vi "Main On Load Action VI.vi"(8 "error in (no error)":errorcluster, 11 "Device Item Ref in":T1 format="%.0x") -> (0 "error out":errorcluster, 3 "Device Item Ref out":T1 format="%.0x")   [LabVIEW 2019, in "Engine Simulation Toolkit System Explorer.lvlib"]
uses:
  Engine Simulation Toolkit System Explorer.lvlib
  <vilib>/NI VeriStand/Custom Device API/Custom Device Item Ref.ctl
  NationalInstruments.VeriStand.SystemDefinitionAPI
  Shared/Constants and GUIDs.vi
  <vilib>/NI VeriStand/Custom Device API/Custom Device API.lvlib
  Shared/Engine Simulation Toolkit Shared.lvlib
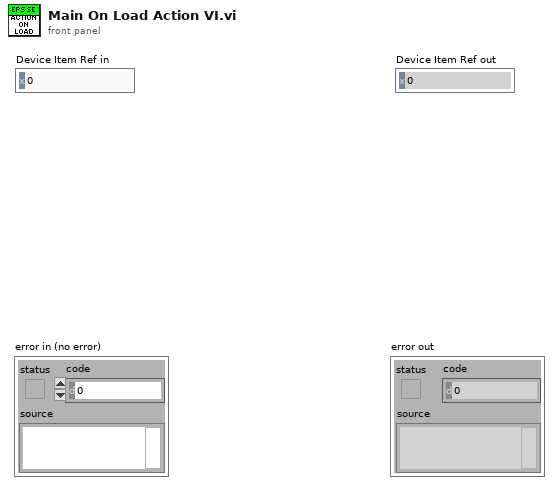
[diagram p1: front panel]
types:
  T1 = typedef "Custom Device API.lvlib/Custom Device Item Ref.ctl" = u64
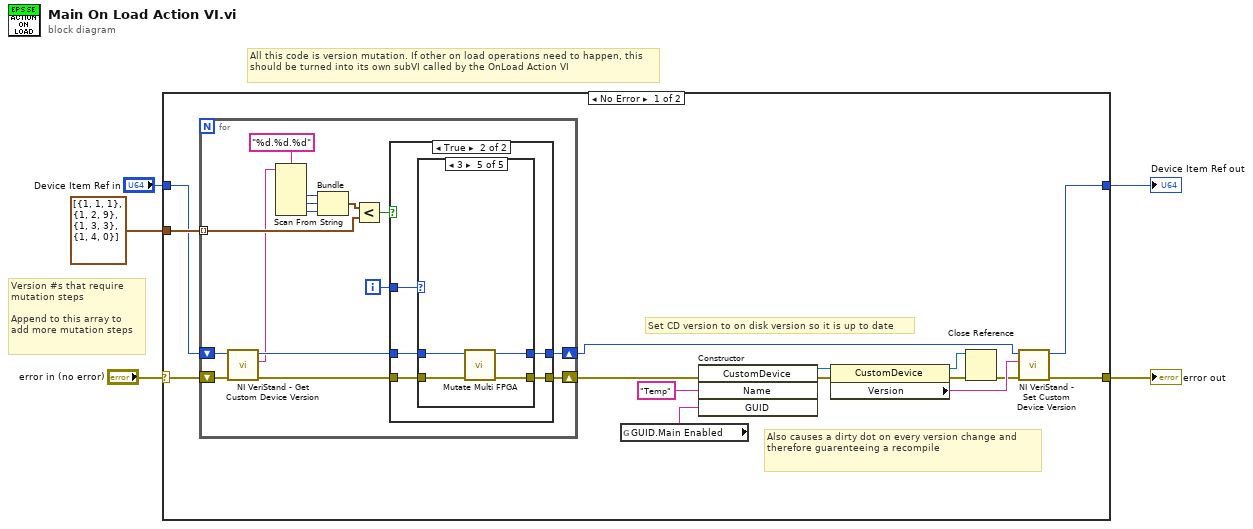
[diagram p0: block diagram]
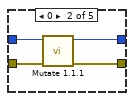
[diagram p4: hidden frame]
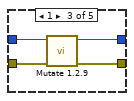
[diagram p5: hidden frame]
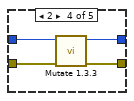
[diagram p6: hidden frame]
diagram:
  # "All this code is version mutation. If other on load operations need to happen, this should be turned into its own subVI called by the OnLoad Action VI"
  # "Version #s that require\nmutation steps\n\nAppend to this array to\nadd more mutation steps"
  n1 = case shown="No Error" "error in (no error)" {
    selector: "error in (no error)" -> [w19 w62]
    tunnel: [w17 w62] -> w4
    tunnel: "Device Item Ref in" -> [w18 w61]
    tunnel: [w16 w61] -> w2
    tunnel: cluster{i32, i32, i32}[] [{1, 1, 1}, {1, 2, 9}, {1, 3, 3}, {1, 4, 0}] -> [w20 _]
    frame No Error {
      # "Also causes a dirty dot on every version change and therefore guarenteeing a recompile"
      # "Set CD version to on disk version so it is up to date"
      n2 = for {
        tunnel: w20 -> [w23] mode=indexing
        shift-right: [w27] -> w7
        shift-left: w19 -> [w31]
        shift-right: [w25] -> w6
        shift-left: w18 -> [w30]
        i -> [w24]
        n3 = call <vilib>:"NI VeriStand - Get Custom Device Version.vi"("error in (no error)"=w31, "Device Ref in"=w30) -> ("error out"=w28:errorcluster, "Value"=w21:string, "Device Ref out"=w26:T1)  [unwired: 7 in]
        n4 = Scan From String(format string="%d.%d.%d", input string=w21) -> (output 1=w33:i32, output 2=w34:i32, output 3=w22:i32)  [unwired: 5 in, 3 out]
        n5 = Bundle(w33, w34, w22) -> (w35:cluster{i32, i32, i32})  [unwired: 1 in]
        n6 = Less?(x=w35, y=w23) -> (x < y?=w29:bool)
        n7 = case shown="True" w29 {
          tunnel: w28 -> [w37 w42]
          tunnel: [w37 w41] -> w27
          tunnel: w26 -> [w36 w38]
          tunnel: [w36 w39] -> w25
          tunnel: w24 -> [_ w40]
          frame False {
          }
          frame True {
            n8 = case shown="3" w40 {
              tunnel: w42 -> [w44 w47 w51 w55 w59]
              tunnel: [w44 w46 w50 w54 w57] -> w41
              tunnel: [w43 w45 w49 w53 w58] -> w39
              tunnel: w38 -> [w43 w48 w52 w56 w60]
              frame Default {
              }
              frame 0 {
                n9 = call "Mutate 1.1.1.vi"("error in (no error)"=w47, "Device Ref in"=w48) -> ("error out"=w46:errorcluster, "Device Ref out"=w45:T1)  [unwired: 8 in]
              }
              frame 1 {
                n10 = call "Mutate 1.2.9.vi"("error in (no error)"=w51, "Device Ref in"=w52) -> ("error out"=w50:errorcluster, "Device Ref out"=w49:T1)  [unwired: 8 in]
              }
              frame 2 {
                n11 = call "Mutate 1.3.3.vi"("error in (no error)"=w55, "Device Ref in"=w56) -> ("error out"=w54:errorcluster, "Device Ref out"=w53:T1)  [unwired: 8 in]
              }
              frame 3 {
                n12 = call "Mutate Multi FPGA.vi"("error in (no error)"=w59, "Device Ref in"=w60) -> ("error out"=w57:errorcluster, "Device Ref out"=w58:T1)  [unwired: 8 in]
              }
            }
          }
        }
      }
      n13 = global read "Constants and GUIDs.vi" "GUID.Main Enabled"() -> (w8:string)
      n14 = constructor class="CustomDevice"(error in=w7, "Name"="Temp", "GUID"=w8) -> (reference out=w14:refnum<k24>, error out=w13:errorcluster)  [unwired: 2 in, 3 out]
      n15 = property class="CustomDevice"(reference=w14, error in=w13) -> (reference out=w11:refnum<k24>, error out=w12:errorcluster, "Version"=w10:string)
      n16 = Close Reference(reference=w11, error in (no error)=w12) -> (error out=w9:errorcluster)
      n17 = call <vilib>:"NI VeriStand - Set Custom Device Version.vi"("error in (no error)"=w9, "Value"=w10, "Device Ref in"=w6) -> ("error out"=w17:errorcluster, "Device Ref out"=w16:T1)  [unwired: 7 in]
    }
    frame Error {
    }
  }
  "error out" <- w4
  "Device Item Ref out" <- w2
